vi "Cleanup.vi"(8 "error in (no error)":errorcluster, 11 "Status in":refnum<class "Status.lvclass">) -> (0 "error out":errorcluster)   [LabVIEW 2020, in "neg-pkg.lvlib" / "Status.lvclass"]
uses:
  Status.lvclass
  Status.lvclass/Status.ctl
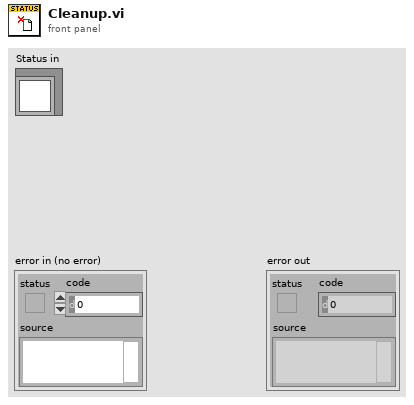
[diagram p1: front panel]
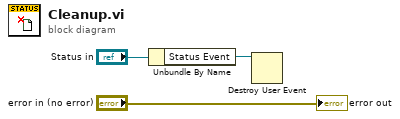
[diagram p0: block diagram]
diagram:
  n1 = Unbundle By Name("Status in") -> ("Status Event"=w1:refnum<user-event>)
  n2 = Destroy User Event(user event=w1) -> ()  [unwired: 1 in, 1 out]
  "error out" <- "error in (no error)"
